vi "0036-Sub_CP2112＿SHT31.vi"(8 "エラー入力（エラーなし）":errorcluster, 10 "アドレス":i32, 11 "device入力":T1) -> (0 "エラー出力":errorcluster, 2 "配列":u8[](array[numeric]), 3 "deviceOut":T1)   [LabVIEW 2014]
uses:
  <userlib>/LV-CP2112_2014/LVProject/private/CP2112_device.ctl
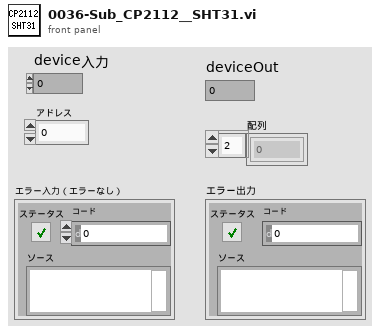
[diagram p1: front panel]
types:
  T1 = typedef "CP2112_device.ctl" = i32
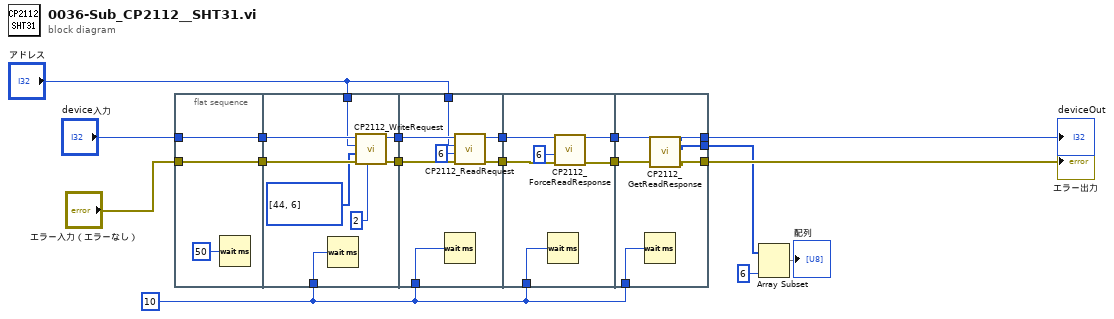
[diagram p0: block diagram]
diagram:
  w3 = u32 10 ("ミリ秒待機時間")
  n1 = flat-sequence {
    tunnel: "device入力" -> [w19]
    tunnel: "エラー入力（エラーなし）" -> [w20]
    tunnel: [w20] -> w2
    tunnel: [w19] -> w1
    tunnel: "アドレス" -> [w22]
    tunnel: [w26] -> w17
    tunnel: [w25] -> w16
    tunnel: w3 -> [w21]
    tunnel: w2 -> [w28]
    tunnel: w1 -> [w27]
    tunnel: w17 -> [w33]
    tunnel: w16 -> [w32]
    tunnel: "アドレス" -> [w30]
    tunnel: w3 -> [w29]
    tunnel: [w34] -> w10
    tunnel: [w31] -> w9
    tunnel: w10 -> [w37]
    tunnel: w9 -> [w38]
    tunnel: [w40] -> w8
    tunnel: [w39] -> w7
    tunnel: w3 -> [w36]
    tunnel: w8 -> [w44]
    tunnel: w7 -> [w45]
    tunnel: w3 -> [w42]
    tunnel: [w47] -> w6
    tunnel: [w46] -> w5
    tunnel: [w43] -> w4
    frame #0 {
      n2 = Wait (ms)(milliseconds to wait=u32 50 ("ミリ秒待機時間")) -> ()  [unwired: 1 out]
    }
    frame #1 {
      n3 = Wait (ms)(milliseconds to wait=w21) -> ()  [unwired: 1 out]
      n4 = call <userlib>:"CP2112_WriteRequest.vi"("numBytesToWrite"=i16 2 ("numByteToRead"), "error in (no error)"=w28, "buffer"=u8[] [44, 6], "slaveAddress"=w22, "device"=w27) -> ("error out"=w26:errorcluster, "deviceOut"=w25:T1)  [unwired: 4 in, 1 out]
    }
    frame #2 {
      n5 = Wait (ms)(milliseconds to wait=w29) -> ()  [unwired: 1 out]
      n6 = call <userlib>:"CP2112_ReadRequest.vi"("error in (no error)"=w33, "numByteToRead"=i16 6, "slaveAddress"=w30, "device"=w32) -> ("error out"=w34:errorcluster, "deviceOut"=w31:T1)  [unwired: 5 in, 1 out]
    }
    frame #3 {
      n7 = Wait (ms)(milliseconds to wait=w36) -> ()  [unwired: 1 out]
      n8 = call <userlib>:"CP2112_ForceReadResponse.vi"("error in (no error)"=w37, "numByteToRead"=i16 6, "device"=w38) -> ("error out"=w40:errorcluster, "deviceOut"=w39:T1)  [unwired: 6 in, 1 out]
    }
    frame #4 {
      n9 = Wait (ms)(milliseconds to wait=w42) -> ()  [unwired: 1 out]
      n10 = call <userlib>:"CP2112_GetReadResponse.vi"("error in (no error)"=w44, "device"=w45) -> ("error out"=w47:errorcluster, "buffer"=w43:u8[], "deviceOut"=w46:T1)  [unwired: 4 in, 3 out]
    }
  }
  n11 = Array Subset(array=w4, length=6 ("長さ")) -> (→"配列":u8[])  [unwired: 1 in]
  "deviceOut" <- w5
  "エラー出力" <- w6
